vi "Set New Value.vi"(8 "Error In":errorcluster, 10 "New Value":dbl, 11 "Graph In":refnum<class "Graph.lvclass">) -> (0 "Error Out":errorcluster, 3 "Graph Out":refnum<class "Graph.lvclass">)   [LabVIEW 2019, in "Graph.lvclass"]
uses:
  Graph.lvclass
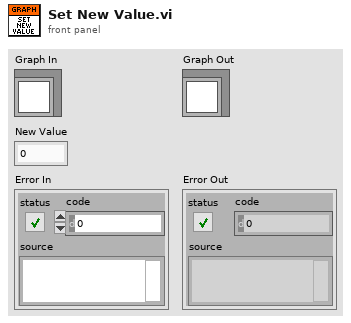
[diagram p1: front panel]
types:
  T1 = typedef "Graph.lvclass/Range.ctl" = cluster{"Maximum":dbl, "Minimum":dbl}
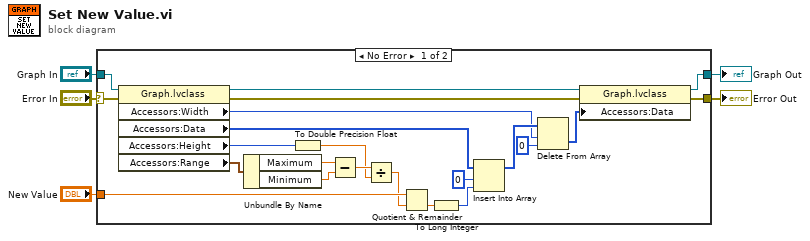
[diagram p0: block diagram]
diagram:
  n1 = case shown="No Error" "Error In" {
    selector: "Error In" -> [w26 w29]
    tunnel: "Graph In" -> [w27 w28]
    tunnel: [w6 w29] -> w3
    tunnel: [w7 w28] -> w2
    tunnel: "New Value" -> [w21 _]
    frame No Error {
      n2 = property class="Graph.lvclass"(reference=w27, error in=w26) -> (reference out=w17:refnum<class "Graph.lvclass">, error out=w16:errorcluster, "Accessors:Width"=w10:u32, "Accessors:Data"=w12:i32[], "Accessors:Height"=w15:u32, "Accessors:Range"=w25:T1)
      n3 = Unbundle By Name(w25) -> ("Maximum"=w24:dbl, "Minimum"=w23:dbl)
      n4 = To Double Precision Float(number=w15) -> (double precision float=w19:dbl)
      n5 = Subtract(x=w24, y=w23) -> (x-y=w22:dbl)
      n6 = Divide(x=w22, y=w19) -> (x/y=w20:dbl)
      n7 = Quotient & Remainder(x=w21, y=w20) -> (floor(x/y)=w18:dbl)  [unwired: 1 out]
      n8 = To Long Integer(number=w18) -> (32bit integer=w14:i32)
      n9 = Insert Into Array(array=w12, index=0, new element=w14) -> (w11:i32[])
      n10 = Delete From Array(array=w11, length=w10, index=0) -> (deleted portion=w8:i32[])  [unwired: 1 out]
      n11 = property class="Graph.lvclass"(reference=w17, error in=w16, "Accessors:Data"=w8) -> (reference out=w7:refnum<class "Graph.lvclass">, error out=w6:errorcluster)
    }
    frame Error {
    }
  }
  "Graph Out" <- w2
  "Error Out" <- w3
